vi "CreateImages.vi"(8 "error in (no error)":errorcluster, 10 "Numeric":i32, 11 "MagSpec_Bella in":refnum<class "MagSpec_Bella.lvclass">) -> (0 "error out":errorcluster, 3 "MagSpec_Bella out":refnum<class "MagSpec_Bella.lvclass">)   [LabVIEW 2013, in "MagSpec_Bella.lvclass"]
uses:
  MagSpec_Bella.lvclass
  MagSpec_Bella.lvclass/MagSpec_Bella.ctl
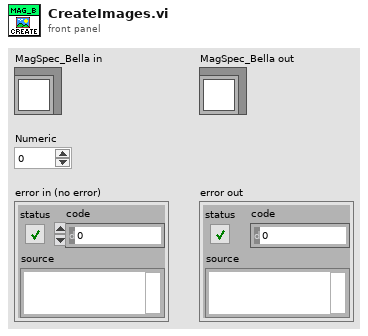
[diagram p1: front panel]
types:
  T1 = typedef "Image Type" = u32
  T2 = typedef "IMAQ Image.ctl" = refnum<image>
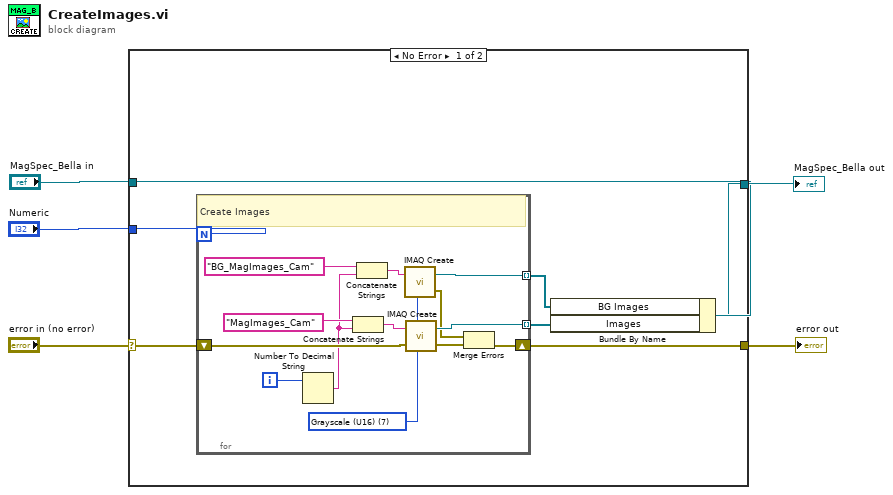
[diagram p0: block diagram]
diagram:
  n1 = case shown="No Error" "error in (no error)" {
    selector: "error in (no error)" -> [w6 w27]
    tunnel: "MagSpec_Bella in" -> [w12 w26]
    tunnel: "Numeric" -> [w11 _]
    tunnel: [w10 w26] -> w3
    tunnel: [w8 w27] -> w2
    frame No Error {
      n2 = for {
        N: w11 -> [_]
        tunnel: [w22] -> w9 mode=indexing
        shift-right: [w13] -> w8
        shift-left: w6 -> [w21]
        tunnel: [w14] -> w7 mode=indexing
        i -> [w25]
        w20 = T1 7 items=["Grayscale (U8)", "Grayscale (I16)", "Grayscale (SGL)", "Complex (CSG)", "RGB (U32)", "HSL (U32)", "RGB (U64)", "Grayscale (U16)"] ("Image Type")
        # "Create Images"
        n3 = Number To Decimal String(number=w25) -> (decimal integer string=w18:string)  [unwired: 1 in]
        n4 = Concatenate Strings("MagImages_Cam" ("string"), w18) -> (w23:string)
        n5 = Concatenate Strings("BG_MagImages_Cam" ("string"), w18) -> (w17:string)
        n6 = call "IMAQ Create"("Image Name"=w17, "Image Type"=w20) -> ("New Image"=w14:T2, "error out"=w16:errorcluster)  [unwired: 3 in]
        n7 = call "IMAQ Create"("Image Name"=w23, "Image Type"=w20, "error in (no error)"=w21) -> ("New Image"=w22:T2, "error out"=w15:errorcluster)  [unwired: 2 in]
        n8 = Merge Errors(w16, w15) -> (w13:errorcluster)
      }
      n9 = Bundle By Name(cluster=w12, "BG Images"=w7, "Images"=w9) -> (w10:refnum<class "MagSpec_Bella.lvclass">)
    }
    frame Error {
    }
  }
  "MagSpec_Bella out" <- w3
  "error out" <- w2
